vi "styleName.vi"(8 "Error In":errorcluster, 11 "QFont In":refnum<class "QFont.lvclass">) -> (0 "Error Out":errorcluster, 2 "Value":string, 3 "QFont Out":refnum<class "QFont.lvclass">)   [LabVIEW 2014, in "QFont.lvclass"]
doc: "LabVIEW-specific documentation is not yet available. See <b>https://doc.qt.io/qt-5/qfont.html#styleName</b>"
uses:
  QFont.lvclass
  LQ Core/LQSerialData/LQSerialData.lvclass/LQSerialData.ctl
  LQ Core/LQ Core.lvlib
  LQ Core/LQSerialData/LQSerialData.lvclass
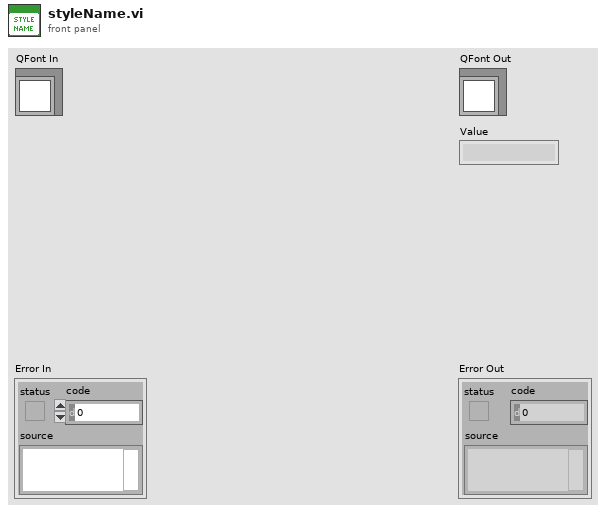
[diagram p1: front panel]
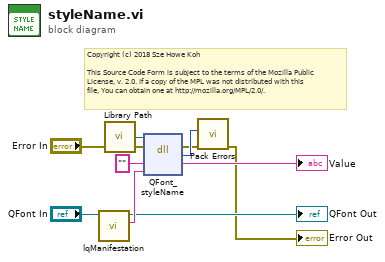
[diagram p0: block diagram]
diagram:
  # "Copyright (c) 2018 Sze Howe Koh\n\nThis Source Code Form is subject to the terms of the Mozilla Public\nLicense, v. 2.0. If a copy of the MPL was not distributed with this\nfile, You can obtain one at http://mozilla.org/MPL/2.0/."
  n1 = call "lqManifestation.vi"("LQSerialData in"="QFont In") -> ("Manifestation"=w7:string, "LQSerialData out"=→"QFont Out":refnum<class "QFont.lvclass">)  [unwired: 9 in]
  n2 = call "Library Path.vi"() -> ("Library Path"=w4:path)
  n3 = dll-call lib="?" fn="QFont_styleName"(path in=w4, error in="Error In", "_retVal"="" ("retVal"), "_instance"=w7) -> (error out=w2:errorcluster, w3:i32, "_retVal"=→"Value":string)  [unwired: 2 in, 1 out]
  n4 = call "Pack Errors.vi"("Error In"=w2, "Error Code"=w3) -> ("Error Out"=→"Error Out":errorcluster)  [unwired: 9 in]
